vi "LinkNodes.vi"(6 "index":i32, 8 "error in":errorcluster, 10 "child in":T1, 11 "parent in":T1) -> (0 "error out":errorcluster, 2 "child out":T1, 3 "parent out":T1)   [LabVIEW 2013, in "NISE_CEF_Node.lvclass"]
doc: "Links 2 nodes together one as a parent and one as a child."
uses:
  NISE_CEF_Node.lvclass
  NodeRef.ctl
  NISE_CEF_Node.lvclass/NISE_CEF_Node.ctl
  ReadChildren.vi
  WriteChildren.vi
  WriteParent.vi
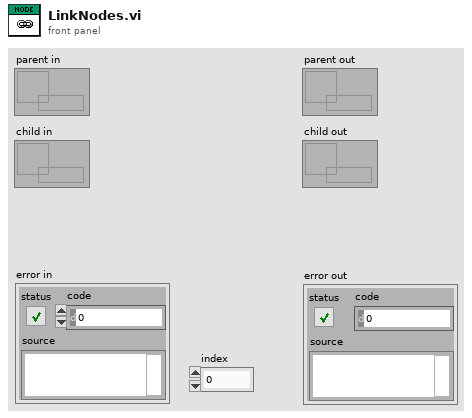
[diagram p1: front panel]
types:
  T1 = typedef "NISE_CEF_Node.lvclass/NodeRef.ctl" = refnum<data-value>
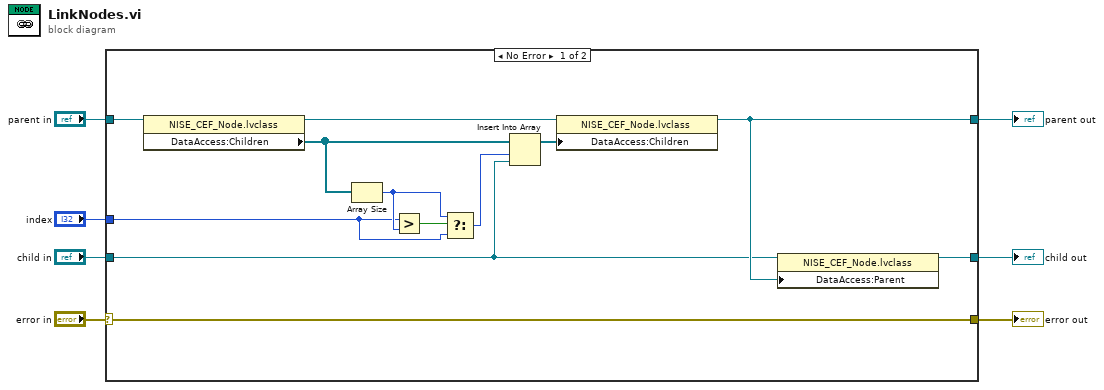
[diagram p0: block diagram]
diagram:
  n1 = case shown="No Error" "error in" {
    selector: "error in" -> [w19 w22]
    tunnel: [w19 w22] -> w3
    tunnel: "parent in" -> [w13 w21]
    tunnel: "child in" -> [w9 w20]
    tunnel: [w8 w20] -> w2
    tunnel: [w11 w21] -> w1
    tunnel: "index" -> [w16 _]
    frame No Error {
      n2 = property class="NISE_CEF_Node.lvclass"(reference=w13) -> (reference out=w10:T1, "DataAccess:Children"=w15:T1[])  [unwired: 1 in, 1 out]
      n3 = Array Size(array=w15) -> (size(s)=w17:i32)
      n4 = Greater?(x=w16, y=w17) -> (0:w18:bool)
      n5 = Select(t=w17, s=w18, f=w16) -> (s? t:f=w14:i32)
      n6 = Insert Into Array(array=w15, index=w14, new element=w9) -> (w12:T1[])
      n7 = property class="NISE_CEF_Node.lvclass"(reference=w10, "DataAccess:Children"=w12) -> (reference out=w11:T1)  [unwired: 1 in, 1 out]
      n8 = property class="NISE_CEF_Node.lvclass"(reference=w9, "DataAccess:Parent"=w11) -> (reference out=w8:T1)  [unwired: 1 in, 1 out]
    }
    frame Error {
    }
  }
  "error out" <- w3
  "child out" <- w2
  "parent out" <- w1
